vi "image.vi"(8 "error in":errorcluster, 11 "Session In":T1) -> (0 "error out":errorcluster, 1 "Inspection Status":bool, 2 "Image":T2(plugin-control))   [LabVIEW 2015]
uses:
  <vilib>/userdefined/High Color/VBAIInterface.ctl
  <vilib>/vision/Vision Builder AI/API.llb/VBAI Interface - Get Inspection Image (By Name).vi
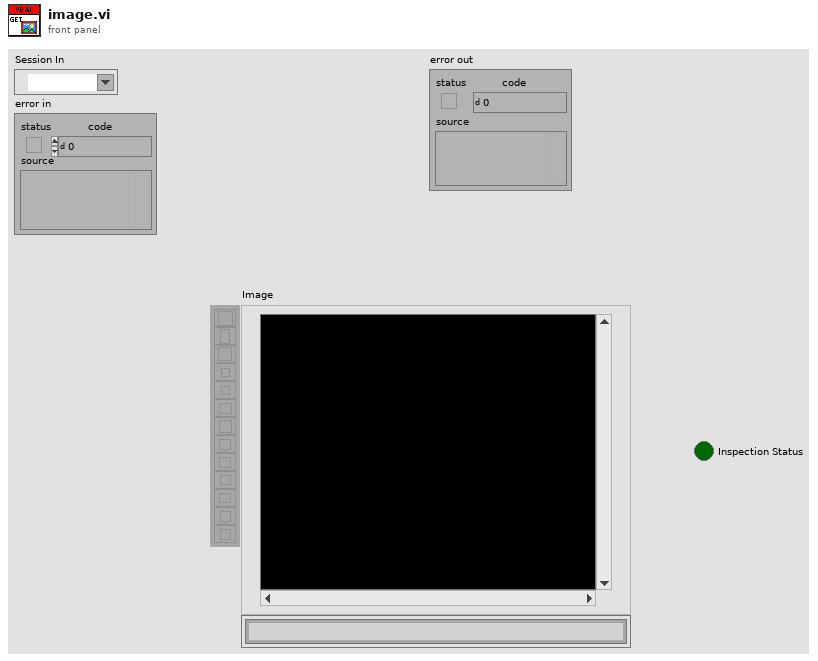
[diagram p1: front panel]
types:
  T1 = typedef "VBAIInterface.ctl" = refnum<k21>
  T2 = typedef "IMAQ Image.ctl" = refnum<image>
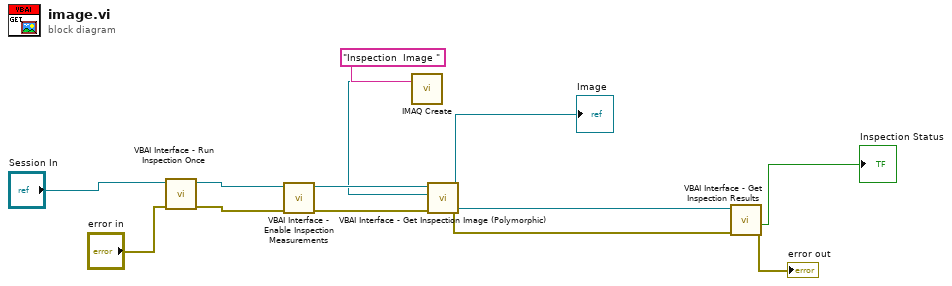
[diagram p0: block diagram]
diagram:
  n1 = call <vilib>:"VBAI Interface - Run Inspection Once.vi"("error in"="error in", "Session In"="Session In") -> ("error out"=w11:errorcluster, "Session Out"=w12:T1)  [unwired: 8 in]
  n2 = call <vilib>:"VBAI Interface - Enable Inspection Measurements.vi"("error in"=w11, "Session In"=w12) -> ("error out"=w9:errorcluster, "Session Out"=w10:T1)  [unwired: 8 in]
  n3 = call "IMAQ Create"("Image Name"="Inspection  Image ") -> ("New Image"=w8:T2)  [unwired: 4 in, 1 out]
  n4 = call-poly <vilib>:"VBAI Interface - Get Inspection Image (Polymorphic).vi"("error in"=w9, "Image Dest"=w8, "Session In"=w10) -> ("error out"=w5:errorcluster, "Image Dst Out"=→"Image":T2, "Session Out"=w6:T1)  [unwired: 5 in, 1 out]
  n5 = call <vilib>:"VBAI Interface - Get Inspection Results.vi"("error in"=w5, "Session In"=w6) -> ("error out"=→"error out":errorcluster, "Inspection Status"=→"Inspection Status":bool)  [unwired: 3 in, 5 out]
